vi "Restore Corrupt Statechart.vi"() -> ()   [LabVIEW 2010]
panel:
  out "error out":errorcluster
  in  "Path to statechart":path
  # "1. Make sure no projects/VIs/statecharts are open except this VI.\n2. Point this VI to your statechart which has a bad CustomDataDisplay.vi.\n3. Run this VI.\n4. Close this VI.\n5. Open your statechart and open CustomDataDisplay.vi. You will get a prompt about the VI not being in the library. Click update.\n6. You may get a dialog complaining about dependencies loaded from unexpected paths. Ignore these.\n6. Save your statechart."
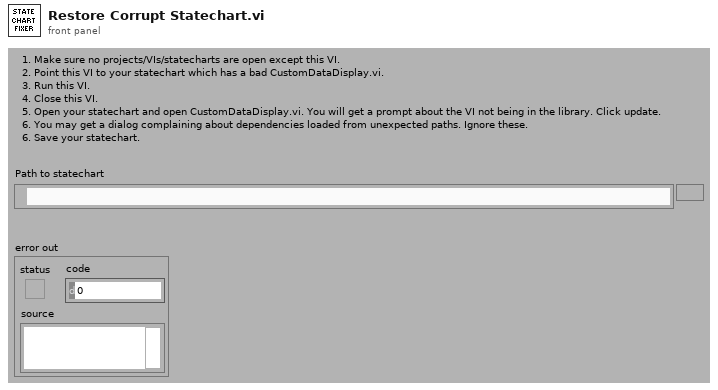
[diagram p1: front panel]
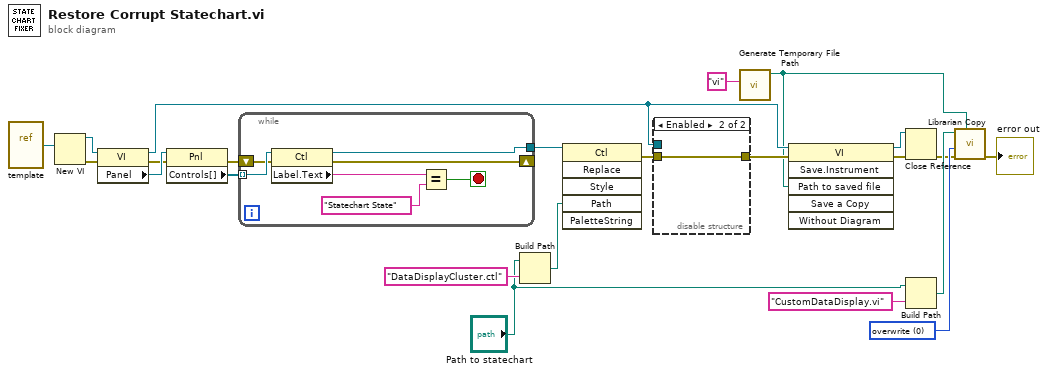
[diagram p0: block diagram]
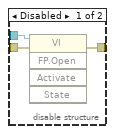
[diagram p2: hidden frame]
diagram:
  w3 = u16 0 items=["overwrite", "ask first", "don't overwrite"] ("overwrite")
  n1 = vi-ref "template.vi"() -> (w22:refnum<vi>)
  n2 = New VI(10:w22) -> (0:w18:errorcluster, 3:w21:refnum<vi>)  [unwired: 6 in]
  n3 = property class="VI"(reference=w21, error in=w18) -> (reference out=w11:refnum<vi>, error out=w17:errorcluster, "Panel"=w20:refnum<vi>)
  n4 = property class="Pnl"(reference=w20, error in=w17) -> (error out=w16:errorcluster, "Controls[]"=w19:refnum<vi>[])  [unwired: 1 out]
  n5 = while {
    tunnel: w19 -> [w30] mode=indexing
    shift-right: [w24] -> _
    shift-left: w16 -> [w29]
    tunnel: [w25] -> w15
    stop <- w26 stop-if-true
    n6 = property class="Ctl"(reference=w30, error in=w29) -> (reference out=w25:refnum<vi>, error out=w24:errorcluster, "Label.Text"=w28:string)
    n7 = Equal?(x=w28, y="Statechart State") -> (x = y?=w26:bool)
  }
  n8 = Build Path(base path="Path to statechart", name or relative path="DataDisplayCluster.ctl") -> (appended path=w14:path)
  n9 = invoke class="Ctl" method="Replace"(reference=w15, "Path"=w14) -> (error out=w13:errorcluster)  [unwired: 4 in, 5 out]
  n10 = disable-structure shown="Enabled" {
    disable-tunnel: w11 -> [w33 _]
    disable-tunnel: w13 -> [w32 w34]
    disable-tunnel: [w31 w34] -> w12
    frame Disabled {
      n11 = invoke class="VI" method="FP.Open"(reference=w33, error in=w32) -> (error out=w31:errorcluster)  [unwired: 3 in, 4 out]
    }
    frame Enabled {
    }
  }
  n12 = call <vilib>:"Generate Temporary File Path.vi"("Temporary File Extension (tmp)"="vi") -> ("Unique Temporary File Path"=w5:path)  [unwired: 9 in, 1 out]
  n13 = invoke class="VI" method="Save.Instrument"(reference=w11, error in=w12, "Path to saved file"=w5) -> (reference out=w6:refnum<vi>, error out=w7:errorcluster)  [unwired: 3 in, 4 out]
  n14 = Close Reference(reference=w6, error in (no error)=w7) -> (error out=w2:errorcluster)
  n15 = Build Path(base path="Path to statechart", name or relative path="CustomDataDisplay.vi") -> (appended path=w4:path)
  n16 = call <vilib>:"Librarian Copy.vi"("source"=w5, "error in (no error)"=w2, "overwrite"=w3, "destination"=w4) -> ("error out"=→"error out":errorcluster)  [unwired: 6 in, 1 out]
